vi "main.vi"() -> ()   [LabVIEW 2025]
panel:
  out "inline":dbl
  out "no inline":dbl
  out "direct":dbl
  out "sum":dbl
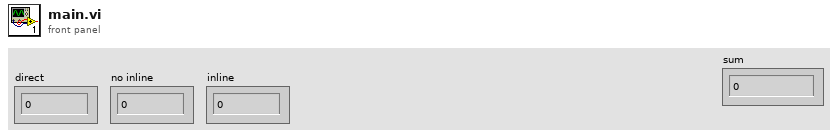
[diagram p1: front panel]
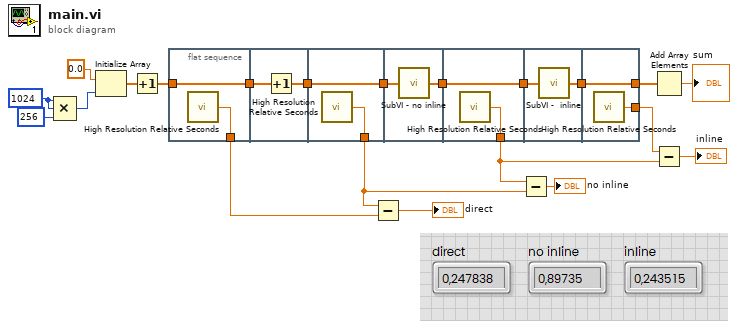
[diagram p0: block diagram]
diagram:
  w19 = 1024
  n1 = Compound Arithmetic op=MULTIPLY(w19, w19, 256 ("value")) -> (w20:i32)
  n2 = Initialize Array(0.0 ("element"), w20) -> (w3:dbl[])
  n3 = Increment(x=w3) -> (x+1=w2:dbl[])
  n4 = flat-sequence {
    tunnel: [w23] -> w18
    tunnel: w2 -> [w23]
    tunnel: [w22] -> w7
    tunnel: w18 -> [w25]
    tunnel: [w24] -> w17
    tunnel: w17 -> [w27]
    tunnel: [w27] -> w16
    tunnel: [w26] -> w8
    tunnel: w16 -> [w29]
    tunnel: [w28] -> w15
    tunnel: w15 -> [w31]
    tunnel: [w31] -> w14
    tunnel: [w30] -> w9
    tunnel: w14 -> [w33]
    tunnel: [w32] -> w13
    tunnel: [w35] -> w12
    tunnel: w13 -> [w35]
    tunnel: [w34] -> w10
    frame #0 {
      n5 = call <vilib>:"High Resolution Relative Seconds.vi"() -> ("relative seconds"=w22:dbl)
    }
    frame #1 {
      n6 = Increment(x=w25) -> (x+1=w24:dbl[])
    }
    frame #2 {
      n7 = call <vilib>:"High Resolution Relative Seconds.vi"() -> ("relative seconds"=w26:dbl)
    }
    frame #3 {
      n8 = call "SubVI - no inline.vi"("Array in"=w29) -> ("Array out"=w28:dbl[])
    }
    frame #4 {
      n9 = call <vilib>:"High Resolution Relative Seconds.vi"() -> ("relative seconds"=w30:dbl)
    }
    frame #5 {
      n10 = call "SubVI -  inline.vi"("Array in"=w33) -> ("Array"=w32:dbl[])
    }
    frame #6 {
      n11 = call <vilib>:"High Resolution Relative Seconds.vi"() -> ("relative seconds"=w34:dbl)
    }
  }
  n12 = Subtract(x=w8, y=w7) -> (x-y=→"direct":dbl)
  n13 = Subtract(x=w9, y=w8) -> (x-y=→"no inline":dbl)
  n14 = Add Array Elements(numeric array=w12) -> (sum=→"sum":dbl)
  n15 = Subtract(x=w10, y=w9) -> (x-y=→"inline":dbl)
